vi "Wall Kick Coordinates.vi"(8 "error in (no error)":errorcluster caption="entrée d'erreur (pas d'erreur)", 10 "New Rotation State":T2, 11 "Piece description":T3) -> (0 "error out":errorcluster caption="sortie d'erreur", 3 "Test Coordinates":T1[](array[typedef]))   [LabVIEW 2017]
uses:
  Controls/Piece Description.ctl
  Controls/Pieces Geometry Names.ctl
  Controls/Coordinates.ctl
  Controls/Rotation State.ctl
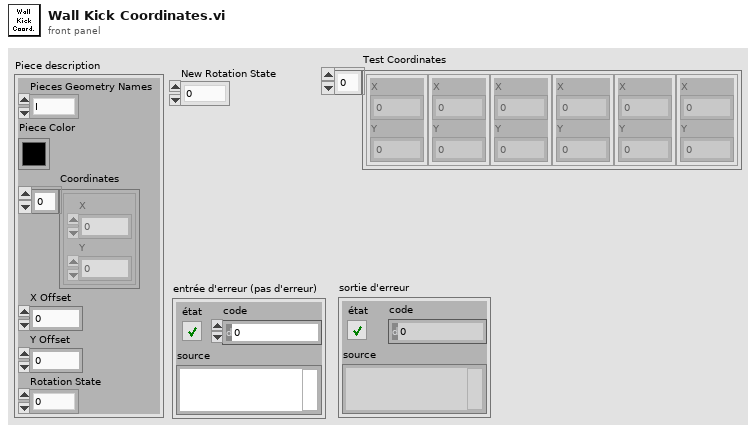
[diagram p1: front panel]
types:
  T1 = typedef "Coordinates.ctl" = cluster{"X":i32, "Y":i32}
  T2 = typedef "Rotation State.ctl" = enum16{"0", "90", "180", "270"}
  T3 = typedef "Piece Description.ctl" = cluster{"Pieces Geometry Names":T4, "Piece Color":u32, "Coordinates":T1[], "X Offset":i32, "Y Offset":i32, "Rotation State":T2}
  T4 = typedef "Pieces Geometry Names.ctl" = enum16{"I", "O", "T", "L", "J", "Z", "S"}
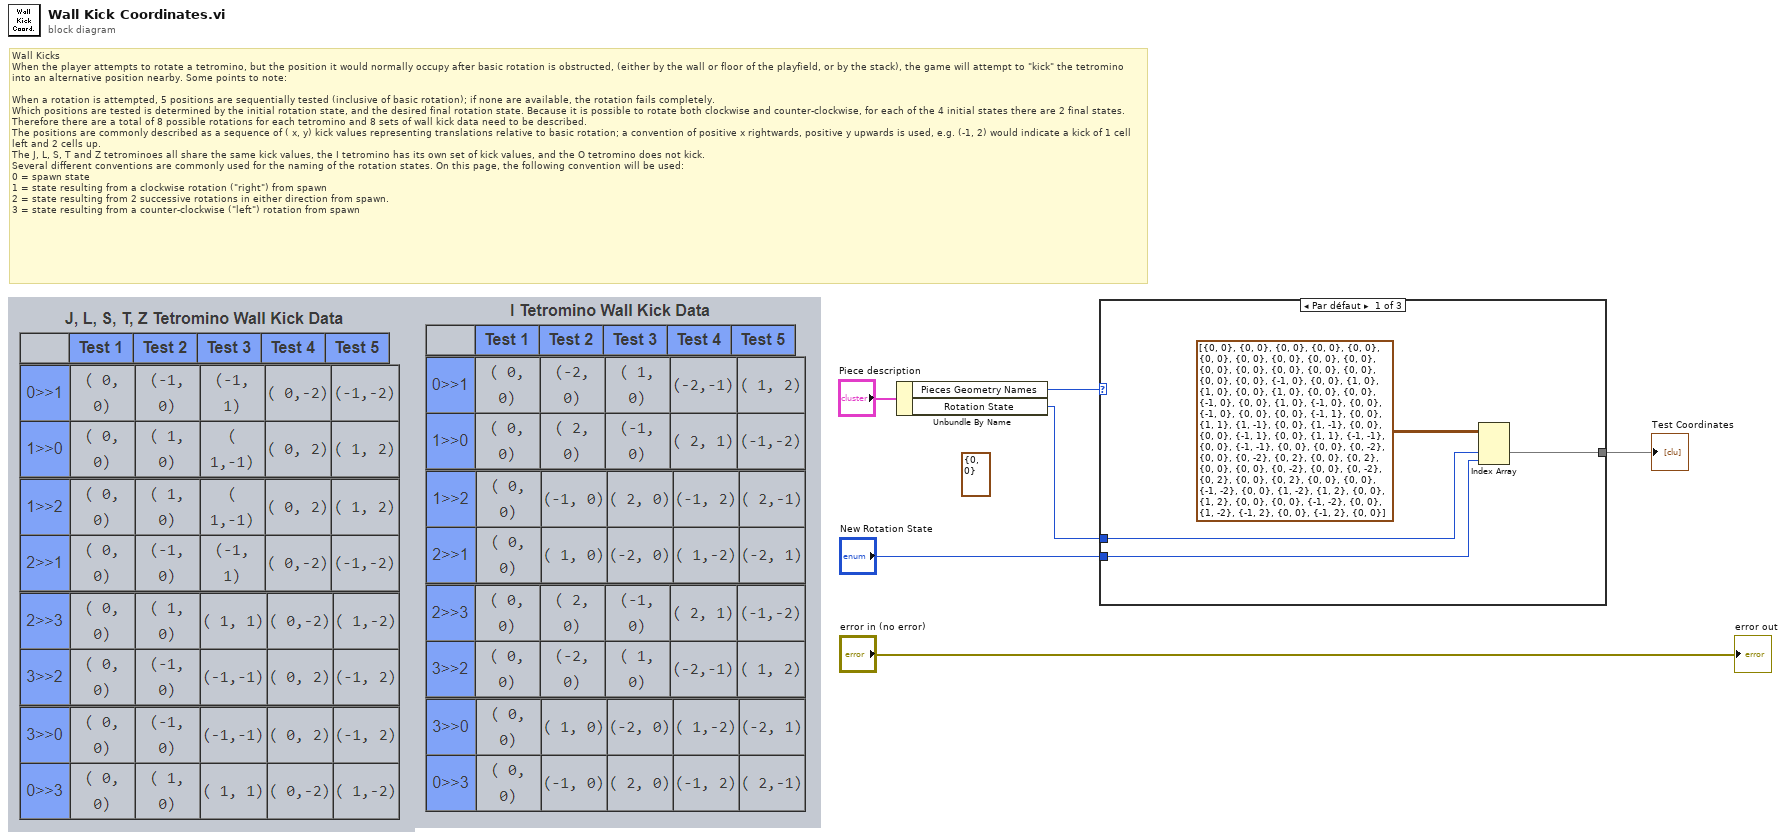
[diagram p0: block diagram]
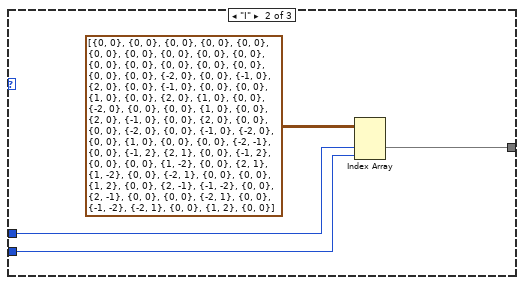
[diagram p2: hidden frame]
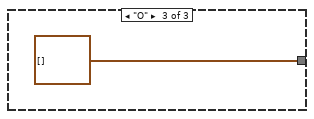
[diagram p3: hidden frame]
diagram:
  (unwired) T1 {"X"=0, "Y"=0} ("Coordinates")
  # "Wall Kicks\nWhen the player attempts to rotate a tetromino, but the position it would normally occupy after basic rotation is obstructed, (either by the wall or floor of the playfield, or by the stack), the game will attempt to \"kick\" the tetromino into an alternative position nearby. Some points to note:\n\nWhen a rotation is attempted, 5 positions are sequentially tested (inclusive of basic rotation); if none are available, the rotation fails completely.\nWhich positions are tested is determined by the initial rotation state, and the desired final rotation state. Because it is possible to rotate both clockwise and counter-clockwise, for each of the 4 initial states there are 2 final states. Therefore there are a total of 8 possible rotations for each tetromino and 8 sets of wall kick data need to be described.\nThe positions are commonly described as a sequence of ( x, y) kick values representing translations relative to basic rotation; a convention of positive x rightwards, positive y upwards is used, e.g. (-1, 2) would indicate a kick of 1 cell left and 2 cells up.\nThe J, L, S, T and Z tetrominoes all share the same kick values, the I tetromino has its own set of kick values, and the O tetromino does not kick.\nSeveral different conventions are commonly used for the naming of the rotation states. On this page, the following convention will be used:\n0 = spawn state\n1 = state resulting from a clockwise rotation (\"right\") from spawn\n2 = state resulting from 2 successive rotations in either direction from spawn.\n3 = state resulting from a counter-clockwise (\"left\") rotation from spawn"
  n1 = Unbundle By Name("Piece description") -> ("Pieces Geometry Names"=w4:T4, "Rotation State"=w3:T2)
  n2 = case shown="Par défaut" w4 {
    tunnel: w3 -> [w8 w13 _]
    tunnel: "New Rotation State" -> [w7 w12 _]
    tunnel: [w9 w11 T1[] [] ("Tableau")] -> w1
    frame Default {
      n3 = Index Array(array=T1[][][] [[[{"X"=0, "Y"=0}, {"X"=0, "Y"=0}, {"X"=0, "Y"=0}, {"X"=0, "Y"=0}], [{"X"=0, "Y"=0}, {"X"=0, "Y"=0}, {"X"=0, "Y"=0}, {"X"=0, "Y"=0}], [{"X"=0, "Y"=0}, {"X"=0, "Y"=0}, {"X"=0, "Y"=0}, {"X"=0, "Y"=0}], [{"X"=0, "Y"=0}, {"X"=0, "Y"=0}, {"X"=0, "Y"=0}, {"X"=0, "Y"=0}]], [[{"X"=0, "Y"=0}, {"X"=-1, "Y"=0}, {"X"=0, "Y"=0}, {"X"=1, "Y"=0}], [{"X"=1, "Y"=0}, {"X"=0, "Y"=0}, {"X"=1, "Y"=0}, {"X"=0, "Y"=0}], [{"X"=0, "Y"=0}, {"X"=-1, "Y"=0}, {"X"=0, "Y"=0}, {"X"=1, "Y"=0}], [{"X"=-1, "Y"=0}, {"X"=0, "Y"=0}, {"X"=-1, "Y"=0}, {"X"=0, "Y"=0}]], [[{"X"=0, "Y"=0}, {"X"=-1, "Y"=1}, {"X"=0, "Y"=0}, {"X"=1, "Y"=1}], [{"X"=1, "Y"=-1}, {"X"=0, "Y"=0}, {"X"=1, "Y"=-1}, {"X"=0, "Y"=0}], [{"X"=0, "Y"=0}, {"X"=-1, "Y"=1}, {"X"=0, "Y"=0}, {"X"=1, "Y"=1}], [{"X"=-1, "Y"=-1}, {"X"=0, "Y"=0}, {"X"=-1, "Y"=-1}, {"X"=0, "Y"=0}]], [[{"X"=0, "Y"=0}, {"X"=0, "Y"=-2}, {"X"=0, "Y"=0}, {"X"=0, "Y"=-2}], [{"X"=0, "Y"=2}, {"X"=0, "Y"=0}, {"X"=0, "Y"=2}, {"X"=0, "Y"=0}], [{"X"=0, "Y"=0}, {"X"=0, "Y"=-2}, {"X"=0, "Y"=0}, {"X"=0, "Y"=-2}], [{"X"=0, "Y"=2}, {"X"=0, "Y"=0}, {"X"=0, "Y"=2}, {"X"=0, "Y"=0}]], [[{"X"=0, "Y"=0}, {"X"=-1, "Y"=-2}, {"X"=0, "Y"=0}, {"X"=1, "Y"=-2}], [{"X"=1, "Y"=2}, {"X"=0, "Y"=0}, {"X"=1, "Y"=2}, {"X"=0, "Y"=0}], [{"X"=0, "Y"=0}, {"X"=-1, "Y"=-2}, {"X"=0, "Y"=0}, {"X"=1, "Y"=-2}], [{"X"=-1, "Y"=2}, {"X"=0, "Y"=0}, {"X"=-1, "Y"=2}, {"X"=0, "Y"=0}]]] ("Tableau"), index (dim 1)=w8, index (dim 2)=w7) -> (element=w9:T1[])  [unwired: 1 in]
    }
    frame "I" {
      n4 = Index Array(array=T1[][][] [[[{"X"=0, "Y"=0}, {"X"=0, "Y"=0}, {"X"=0, "Y"=0}, {"X"=0, "Y"=0}], [{"X"=0, "Y"=0}, {"X"=0, "Y"=0}, {"X"=0, "Y"=0}, {"X"=0, "Y"=0}], [{"X"=0, "Y"=0}, {"X"=0, "Y"=0}, {"X"=0, "Y"=0}, {"X"=0, "Y"=0}], [{"X"=0, "Y"=0}, {"X"=0, "Y"=0}, {"X"=0, "Y"=0}, {"X"=0, "Y"=0}]], [[{"X"=0, "Y"=0}, {"X"=-2, "Y"=0}, {"X"=0, "Y"=0}, {"X"=-1, "Y"=0}], [{"X"=2, "Y"=0}, {"X"=0, "Y"=0}, {"X"=-1, "Y"=0}, {"X"=0, "Y"=0}], [{"X"=0, "Y"=0}, {"X"=1, "Y"=0}, {"X"=0, "Y"=0}, {"X"=2, "Y"=0}], [{"X"=1, "Y"=0}, {"X"=0, "Y"=0}, {"X"=-2, "Y"=0}, {"X"=0, "Y"=0}]], [[{"X"=0, "Y"=0}, {"X"=1, "Y"=0}, {"X"=0, "Y"=0}, {"X"=2, "Y"=0}], [{"X"=-1, "Y"=0}, {"X"=0, "Y"=0}, {"X"=2, "Y"=0}, {"X"=0, "Y"=0}], [{"X"=0, "Y"=0}, {"X"=-2, "Y"=0}, {"X"=0, "Y"=0}, {"X"=-1, "Y"=0}], [{"X"=-2, "Y"=0}, {"X"=0, "Y"=0}, {"X"=1, "Y"=0}, {"X"=0, "Y"=0}]], [[{"X"=0, "Y"=0}, {"X"=-2, "Y"=-1}, {"X"=0, "Y"=0}, {"X"=-1, "Y"=2}], [{"X"=2, "Y"=1}, {"X"=0, "Y"=0}, {"X"=-1, "Y"=2}, {"X"=0, "Y"=0}], [{"X"=0, "Y"=0}, {"X"=1, "Y"=-2}, {"X"=0, "Y"=0}, {"X"=2, "Y"=1}], [{"X"=1, "Y"=-2}, {"X"=0, "Y"=0}, {"X"=-2, "Y"=1}, {"X"=0, "Y"=0}]], [[{"X"=0, "Y"=0}, {"X"=1, "Y"=2}, {"X"=0, "Y"=0}, {"X"=2, "Y"=-1}], [{"X"=-1, "Y"=-2}, {"X"=0, "Y"=0}, {"X"=2, "Y"=-1}, {"X"=0, "Y"=0}], [{"X"=0, "Y"=0}, {"X"=-2, "Y"=1}, {"X"=0, "Y"=0}, {"X"=-1, "Y"=-2}], [{"X"=-2, "Y"=1}, {"X"=0, "Y"=0}, {"X"=1, "Y"=2}, {"X"=0, "Y"=0}]]] ("Tableau"), index (dim 1)=w13, index (dim 2)=w12) -> (element=w11:T1[])  [unwired: 1 in]
    }
    frame "O" {
    }
  }
  "Test Coordinates" <- w1
  "error out" <- "error in (no error)"
